vi "Read Send Data Event.vi"(8 "error in (no error)":errorcluster, 11 "NodeRed-LV-Interface in":refnum<class "NodeRed-LV-Interface.lvclass">) -> (0 "error out":errorcluster, 2 "Send data":refnum<user-event>, 3 "NodeRed-LV-Interface out":refnum<class "NodeRed-LV-Interface.lvclass">)   [LabVIEW 2020, in "NodeRed-LV-Interface.lvclass"]
uses:
  NodeRed-LV-Interface.lvclass
  NodeRed-LV-Interface.lvclass/NodeRed-LV-Interface.ctl
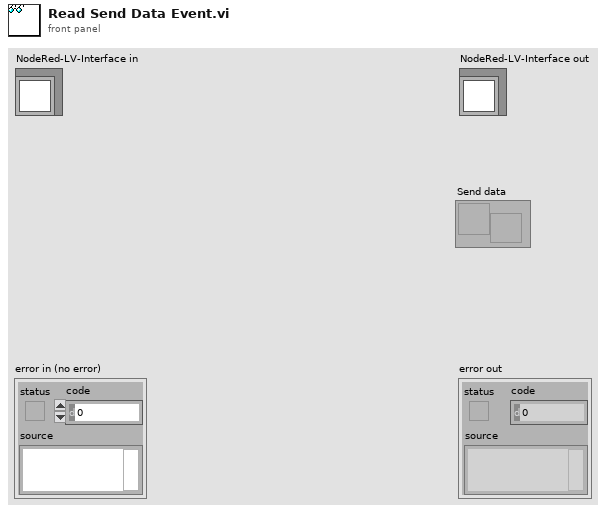
[diagram p1: front panel]
types:
  T1 = cluster{"Send data":refnum<user-event>, "Receive data":refnum<user-event>, "IP Address":string, "Port":u16, "Stop Event":refnum<user-event>, "UDP Engine":refnum<vi>}
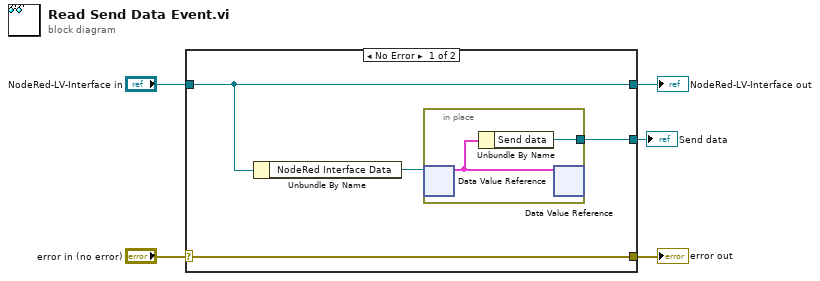
[diagram p0: block diagram]
diagram:
  n1 = case shown="No Error" "error in (no error)" {
    selector: "error in (no error)" -> [w9 w12]
    tunnel: [w9 w12] -> w4
    tunnel: [w8 w13] -> w2
    tunnel: "NodeRed-LV-Interface in" -> [w8 w13]
    tunnel: [w6 _] -> w1
    frame No Error {
      n2 = Unbundle By Name(w8) -> ("NodeRed Interface Data"=w7:refnum<data-value>)
      n3 = in-place {
        in-place-border: [w10] -> w6
        n4 = in-place-dvr #1(w7) -> (w11:T1)  [unwired: 1 out]
        n5 = Unbundle By Name(w11) -> ("Send data"=w10:refnum<user-event>)
        n6 = in-place-dvr #1(w11) -> ()  [unwired: 2 out]
      }
    }
    frame Error {
    }
  }
  "error out" <- w4
  "NodeRed-LV-Interface out" <- w2
  "Send data" <- w1
